vi "Wiimote Loop (Kyle Green's conflicted copy 2012-06-09).vi"() -> ()   [LabVIEW 2011]
doc: "This vi connects to a Wiimote via Bluetooth and passes the necessary controls to the \"Remote\" variables.\nSee Block Diagram:\n1: Open the Wiimote and acquire the device index \n2: Acquire initial calibration data\n3: Get Wiimote sensor data\n4: Set the Trigger enable condition and pass along the XY data\n5: Use a running average to smooth out the control\n6: Apply expo weight for less sensitive control and zero out dead stick offset \n7: Set XY data\n8: XY plot is data binding to network variable for the XY plot on HUD from the Remote tab\n9: Use a stop button titled \"stop?\" so that the LabVIEW script can stop the vi\n10: Close the Wiimote connection\n-Ruffin"
uses:
  <vilib>/Platform/TimedLoop/XDataNode/timing_clust.ctl
  <vilib>/Platform/TimedLoop/XDataNode/nitl_modes.ctl
  <vilib>/Platform/TimedLoop/XDataNode/wakeup.ctl
  <vilib>/Platform/TimedLoop/XDataNode/XDataNode.xnode
  Wiimote.lvlib
  <vilib>/Platform/TimedLoop/XDataNode/XDNodeRunTimeDep.lvlib
panel:
  in  "Expo %":i32(slide)=1 scale=0.0..100.0
  out "Analog Stick":cluster{dbl, dbl}[](graph)
  out "error out":errorcluster
  in  "stop?":bool
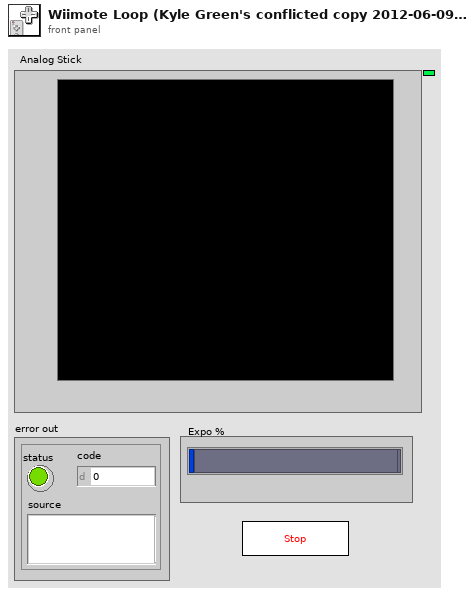
[diagram p1: front panel]
types:
  T1 = typedef "Wiimote.lvlib/Wiimote Acceleration.ctl" = cluster{"Acceleration X":dbl, "Acceleration Y":dbl, "Acceleration Z":dbl}
  T2 = cluster{"Wiimote 0G Calibration":T1, "Wiimote 1G Calibration":T1, "Nunchuk 0G Calibration":T1, "Nunchuk 1G Calibration":T1}
  T3 = typedef "XDNodeRunTimeDep.lvlib/timing_clust.ctl" = cluster{"Expected End [f-1]":u64, "Actual End [f-1]":u64, "Finished Late? [f-1]":bool, "Expected End [i-1]":u64, "Actual End [i-1]":u64, "Finished Late? [i-1]":bool, "Expected Start [i]":u64, "Actual Start [i]":u64, "Expected Start [f]":u64, "Actual Start [f]":u64, "Source Name":string, "Structure Name":string, "Period":i64, "Deadline":i64, "Offset":i64, "Start":i64, "Priority":i32, "Timeout":i32, "Mode":T4, "Wakeup Reason":T5, "Error":errorcluster, "Source Type":string, "Secondary Source Type":string, "Global End Time":u64, "Global Start Time":u64, "Frame Duration":u64, "Iteration Duration":u64, "Assigned CPU":i32, "I/O Scan Engine Mode":u32}
  T4 = typedef "XDNodeRunTimeDep.lvlib/nitl_modes.ctl" = enum32{"No Change", "Process missed periods, maintain original phase", "Discard missed periods, maintain original phase", "Process missed periods, ignore original phase", "Discard missed periods, ignore original phase"}
  T5 = typedef "XDNodeRunTimeDep.lvlib/wakeup.ctl" = enum32{"Normal", "Aborted", "Asynchronous wakeup", "Timing source error", "Timed loop error", "Timeout"}
  T6 = typedef "Wiimote.lvlib/Wiimote Point.ctl" = cluster{"X":u16, "Y":u16}
  T7 = typedef "Wiimote.lvlib/Wiimote Buttons.ctl" = cluster{"D-Pad Left":bool, "D-Pad Right":bool, "D-Pad Down":bool, "D-Pad Up":bool, "Plus":bool, "Two":bool, "One":bool, "B":bool, "A":bool, "Minus":bool, "Home":bool}
  T8 = typedef "Wiimote.lvlib/Nunchuk Buttons.ctl" = cluster{"C":bool, "Z":bool}
  T9 = cluster{"Acceleration Calibrated Out":T1, "Acceleration Calibrated Out":T1, T6[], "Wiimote Buttons":T7, "Nunchuk Buttons":T8, "Nunchuk Analog Stick":cluster{"X":dbl, "Y":dbl}}
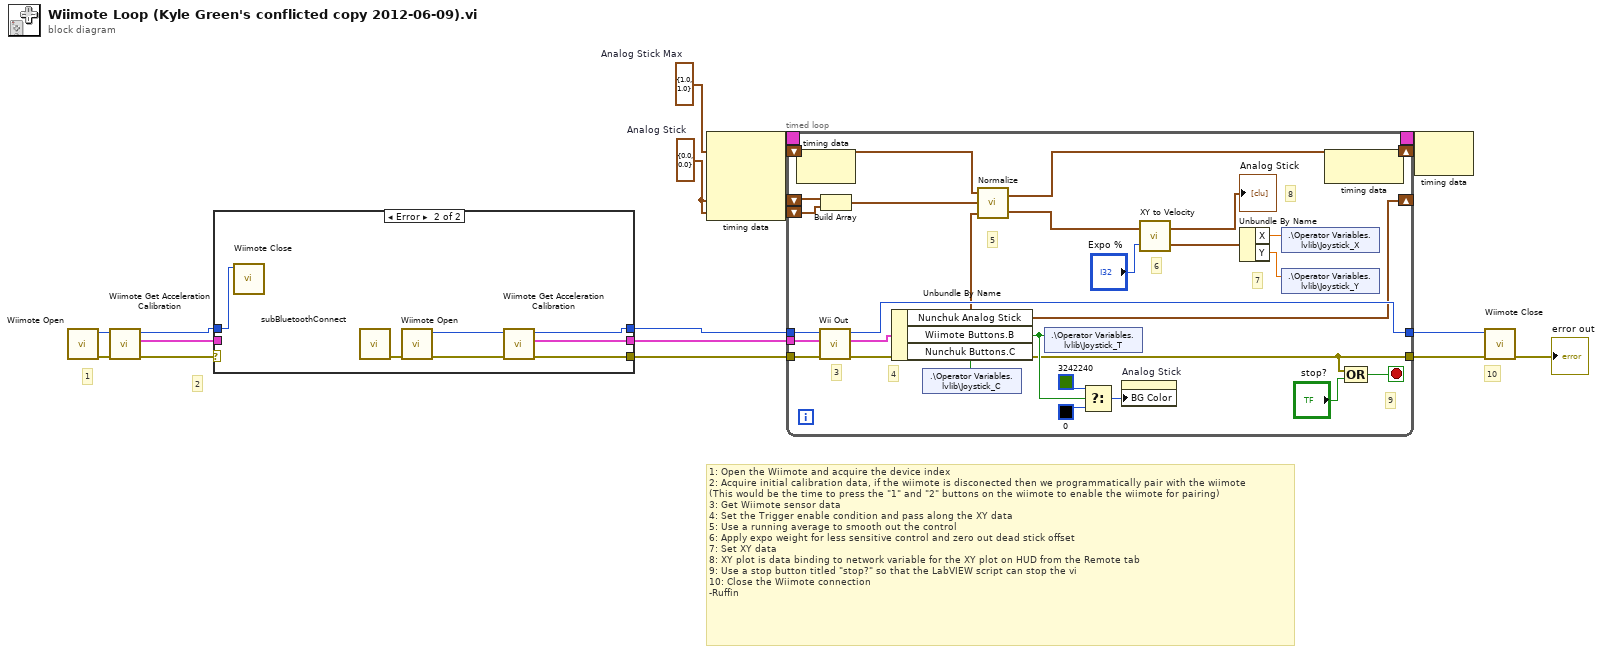
[diagram p0: block diagram]
diagram:
  w12 = cluster{"X":dbl, "Y":dbl} {"X"=1.0, "Y"=1.0}  # Analog Stick Max
  w11 = cluster{"X":dbl, "Y":dbl} {"X"=0.0, "Y"=0.0}  # Analog Stick
  # "2"
  # "1:\tOpen the Wiimote and acquire the device index \n2:\tAcquire initial calibration data, if the wiimote is disconected then we programmatically pair with the wiimote\n(This would be the time to press the \"1\" and \"2\" buttons on the wiimote to enable the wiimote for pairing) \n3:\tGet Wiimote sensor data\n4:\tSet the Trigger enable condition and pass along the XY data\n5:\tUse a running average to smooth out the control\n6:\tApply expo weight for less sensitive control and zero out dead stick offset \n7:\tSet XY data\n8:\tXY plot is data binding to network variable for the XY plot on HUD from the Remote tab\n9:\tUse a stop button titled \"stop?\" so that the LabVIEW script can stop the vi\n10:\tClose the Wiimote connection\n-Ruffin"
  # "10"
  # "1"
  n1 = call "Wiimote Open.vi"() -> ("error out"=w8:errorcluster, "hWiimoteHandle"=w7:u32)  [unwired: 10 in]
  n2 = call "Wiimote Get Acceleration Calibration.vi"("error in"=w8, "hWiimoteHandle in"=w7) -> ("error out"=w1:errorcluster, "Calibration Data Out"=w2:T2, "hWiimoteHandle out"=w3:u32)  [unwired: 7 in]
  n3 = case shown="Error" w1 {
    selector: w1 -> [w18 _]
    tunnel: [w18 w21] -> w5
    tunnel: [w17 w22] -> w6
    tunnel: [w16 w20] -> w4
    tunnel: w3 -> [w17 w19]
    tunnel: w2 -> [w16 _]
    frame No Error {
    }
    frame Error {
      n4 = call "Wiimote Close.vi"("hWiimoteHandle in"=w19) -> ()  [unwired: 10 in, 1 out]
      n5 = call "subBluetoothConnect.vi"() -> ("error out"=w25:errorcluster)  [unwired: 9 in, 2 out]
      n6 = call "Wiimote Open.vi"("error in"=w25) -> ("error out"=w23:errorcluster, "hWiimoteHandle"=w24:u32)  [unwired: 9 in]
      n7 = call "Wiimote Get Acceleration Calibration.vi"("error in"=w23, "hWiimoteHandle in"=w24) -> ("error out"=w21:errorcluster, "Calibration Data Out"=w20:T2, "hWiimoteHandle out"=w22:u32)  [unwired: 7 in]
    }
  }
  n8 = node-c288() -> (w10:T3)  [unwired: 4 in]
  n9 = timed-loop {
    tunnel: w5 -> [w50]
    tunnel: w4 -> [w49]
    tunnel: w6 -> [w48]
    tunnel: [w47] -> w15
    tunnel: [w26] -> w13
    shift-right: [w33] -> _
    shift-left: w11 -> [w36]
    shift-right: [w37] -> _
    shift-left: w12 -> [w38]
    shift-left: w11 -> [w35]
    timing: w10 -> [_]
    timing-out: [_] -> w9
    stop <- w44 stop-if-true
    # "9"
    # "8"
    # "7"
    # "6"
    # "5"
    # "4"
    # "3"
    n10 = node-c288() -> ()  [unwired: 1 in, 1 out]
    n11 = call "Wii Out.vi"("error in"=w50, "Calibration Data In"=w49, "index"=w48) -> ("error out"=w26:errorcluster, "Wii output cluster"=w46:T9, "hWiimoteHandle out"=w47:u32)  [unwired: 2 in]
    n12 = Build Array(w36, w35) -> (w34:cluster{"X":dbl, "Y":dbl}[])
    n13 = Unbundle By Name(w46) -> ("Nunchuk Analog Stick"=w33:cluster{"X":dbl, "Y":dbl}, "Wiimote Buttons.B"=w28:bool, "Nunchuk Buttons.C"=w27:bool)
    n14 = shared-variable ".\\Operator Variables.lvlib\\Joystick_C"(w27) -> ()  [unwired: 1 in, 1 out]
    n15 = call "Normalize.vi"("Analog Stick"=w33, "Past Analog Stick"=w34, "Analog Stick Max"=w38) -> ("Normalized Analog Stick Out"=w32:cluster{"X":dbl, "Y":dbl}, "Analog Stick Max Out"=w37:cluster{"X":dbl, "Y":dbl})
    n16 = shared-variable ".\\Operator Variables.lvlib\\Joystick_T"(w28) -> ()  [unwired: 1 in, 1 out]
    n17 = Select(t=u32 3242240, s=w28, f=u32 0) -> (s? t:f=w29:u32)
    n18 = property on="Analog Stick" class="XYGraph (strict)"("BG Color"=w29) -> ()  [unwired: 2 in, 2 out]
    n19 = call "XY to Velocity.vi"("Expo"="Expo %", "Nunchuk Analog Stick In"=w32) -> ("X and Y"=w41:cluster{"X":dbl, "Y":dbl}, "Nunchuk Analog Stick"=→"Analog Stick":cluster{dbl, dbl}[])
    n20 = Unbundle By Name(w41) -> ("X"=w40:dbl, "Y"=w39:dbl)
    n21 = shared-variable ".\\Operator Variables.lvlib\\Joystick_X"(w40) -> ()  [unwired: 1 in, 1 out]
    n22 = shared-variable ".\\Operator Variables.lvlib\\Joystick_Y"(w39) -> ()  [unwired: 1 in, 1 out]
    n23 = node-c288() -> ()  [unwired: 1 in, 1 out]
    n24 = Compound Arithmetic op=OR(w26, "stop?") -> (w44:bool)
  }
  n25 = node-c288(w9) -> ()  [unwired: 1 out]
  n26 = call "Wiimote Close.vi"("error in"=w13, "hWiimoteHandle in"=w15) -> ("error out"=→"error out":errorcluster)  [unwired: 9 in]
